vi "Script_Create Fixed Wheel.vi"(6 "error source terminal refnum":refnum<vi>, 8 "error in (no error)":errorcluster, 10 "owner diagram refnum":refnum<vi>, 11 "wheel in":refnum<class "NI_Robotics_Wheel.lvclass">) -> (0 "error out":errorcluster, 1 "created?":bool, 2 "wheel out terminal refnum":refnum<vi>, 4 "error out terminal refnum":refnum<vi>)   [LabVIEW 2017, in "NI_Robotics_Scripting Utilities.lvlib"]
uses:
  <vilib>/robotics/Utilities/Scripting/NI_Robotics_Scripting Utilities.lvlib
  <vilib>/robotics/Steering/Wheel/NI_Robotics_Wheel.lvclass
  <vilib>/Utility/miscctls.llb/LVPointTypeDef.ctl
  <vilib>/robotics/Steering/Fixed Wheel/Create Fixed Wheel.vi
  <vilib>/robotics/Steering/Fixed Wheel/NI_Robotics_Fixed Wheel.lvclass
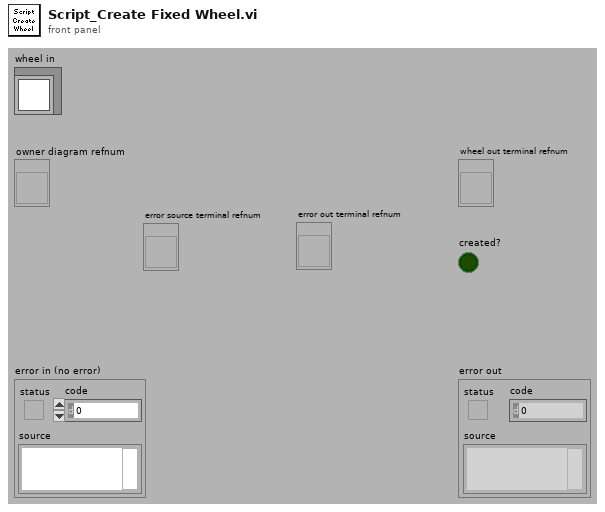
[diagram p1: front panel]
types:
  T1 = typedef "LVPointTypeDef.ctl" = cluster{"Horizontal":i16, "Vertical":i16}
  T2 = typedef "NI_Robotics_Wheel.lvclass/Wheel Parameters.ctl" = cluster{"wheel radius":dbl, "gear ratio":dbl, "forward rotation direction":T3}
  T3 = typedef "NI_Robotics_Wheel.lvclass/Rotation Direction.ctl" = u16
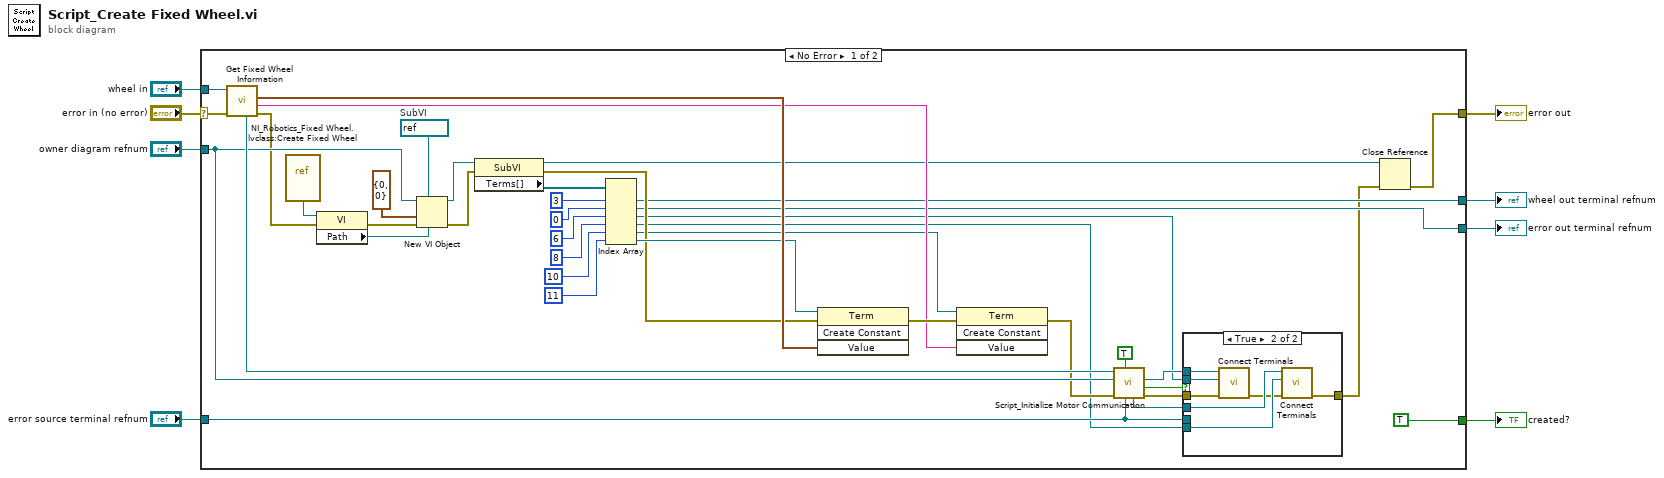
[diagram p0: block diagram]
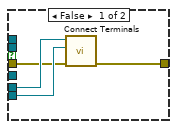
[diagram p2: hidden frame]
diagram:
  n1 = case shown="No Error" "error in (no error)" {
    selector: "error in (no error)" -> [w47 w60]
    tunnel: "wheel in" -> [w48 _]
    tunnel: [w11 w60] -> w6
    tunnel: "owner diagram refnum" -> [w38 _]
    tunnel: [w14 _] -> w4
    tunnel: [w12 _] -> w3
    tunnel: [TRUE _] -> w2
    tunnel: "error source terminal refnum" -> [w28 _]
    frame No Error {
      w44 = refnum<vi> refnum  # SubVI
      n2 = call <vilib>:"Get Fixed Wheel Information.vi"("error in (no error)"=w47, "wheel in"=w48) -> ("error out"=w34:errorcluster, "wheel name"=w36:string, "wheel parameters"=w37:T2, "motor communication"=w46:refnum<class "NI_Robotics_Motor Communication.lvclass">)  [unwired: 5 in, 1 out]
      n3 = vi-ref "NI_Robotics_Fixed Wheel.lvclass:Create Fixed Wheel.vi"() -> (w39:refnum<vi>)
      n4 = property class="VI"(reference=w39, error in=w34) -> (error out=w43:errorcluster, "Path"=w40:path)  [unwired: 1 out]
      n5 = New VI Object(vi object class=w44, owner refnum=w38, position/next to=T1 {"Horizontal"=0, "Vertical"=0} ("relative position/next to refnum"), 6:w40, 8:w43) -> (object refnum=w27:refnum<vi>, 0:w23:errorcluster)  [unwired: 3 in]
      n6 = property class="SubVI"(reference=w27, error in=w23) -> (reference out=w9:refnum<vi>, error out=w22:errorcluster, "Terms[]"=w26:refnum<vi>[])
      n7 = Index Array(array=w26, index #1=3 ("index"), index #2=0 ("index"), index #3=6 ("index"), index #4=8 ("index"), index #5=10 ("index"), index #6=11 ("index")) -> (element #1=w12:refnum<vi>, element #2=w14:refnum<vi>, element #3=w16:refnum<vi>, element #4=w18:refnum<vi>, element #5=w20:refnum<vi>, element #6=w24:refnum<vi>)
      n8 = invoke class="Term" method="Create Constant"(reference=w24, error in=w22, "Value"=w37) -> (error out=w41:errorcluster)  [unwired: 1 in, 3 out]
      n9 = invoke class="Term" method="Create Constant"(reference=w20, error in=w41, "Value"=w36) -> (error out=w30:errorcluster)  [unwired: 1 in, 3 out]
      n10 = call <vilib>:"Script_Initialize Motor Communication.vi"("error source terminal refnum"=w28, "skip if name is empty (F)"=TRUE, "error in (no error)"=w30, "owner diagram refnum"=w38, "motor communication in"=w46) -> ("error out"=w32:errorcluster, "created?"=w33:bool, "motor communication out terminal refnum"=w35:refnum<vi>, "error out terminal refnum"=w31:refnum<vi>)  [unwired: 2 in, 1 out]
      n11 = case shown="True" w33 {
        tunnel: w35 -> [_ w56]
        tunnel: w32 -> [w50 w59]
        tunnel: w31 -> [_ w58]
        tunnel: w18 -> [w51 w57]
        tunnel: [w49 w54] -> w10
        tunnel: w28 -> [w52 _]
        tunnel: w16 -> [_ w53]
        frame False {
          n12 = call <vilib>:"Connect Terminals.vi"("error in (no error)"=w50, "sink terminal"=w51, "source terminal"=w52) -> ("error out"=w49:errorcluster)  [unwired: 7 in, 1 out]
        }
        frame True {
          n13 = call <vilib>:"Connect Terminals.vi"("error in (no error)"=w59, "sink terminal"=w53, "source terminal"=w56) -> ("error out"=w55:errorcluster)  [unwired: 7 in, 1 out]
          n14 = call <vilib>:"Connect Terminals.vi"("error in (no error)"=w55, "sink terminal"=w57, "source terminal"=w58) -> ("error out"=w54:errorcluster)  [unwired: 7 in, 1 out]
        }
      }
      n15 = Close Reference(reference=w9, error in (no error)=w10) -> (error out=w11:errorcluster)
    }
    frame Error {
    }
  }
  "error out" <- w6
  "wheel out terminal refnum" <- w3
  "error out terminal refnum" <- w4
  "created?" <- w2
